vi "Class to Variant.vi"(8 "error in (no error)":errorcluster, 10 "Data in":variant, 11 "Run VI Node in":refnum<class "Run VI Node.lvclass">) -> (0 "error out":errorcluster, 1 "Serialized Object Name":string, 2 "Data":variant, 3 "Run VI Node out":refnum<class "Run VI Node.lvclass">)   [LabVIEW 2014, in "Run VI Node.lvclass"]
uses:
  Run VI Node.lvclass
  Shared/Controls/Run VI - STYP.ctl
  Run VI Node.lvclass/Run VI Node.ctl
  Classes/Build Job/Build Job.lvclass
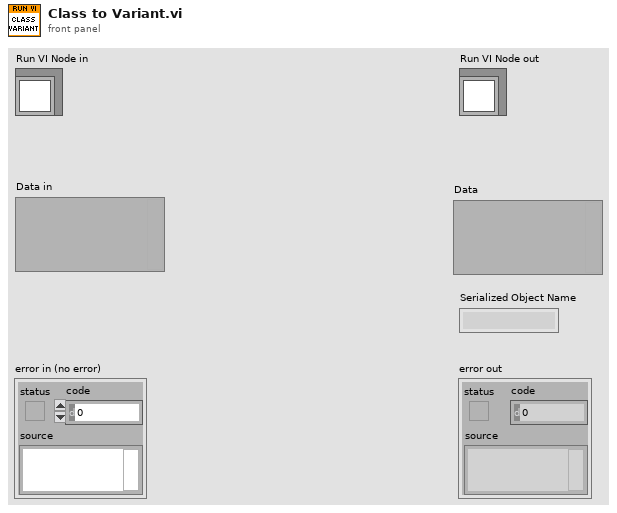
[diagram p1: front panel]
types:
  T1 = typedef "Run VI - STYP.ctl" = cluster{"Executor_Number":string, "VI_Path":string, "Wait_Until_Done":bool}
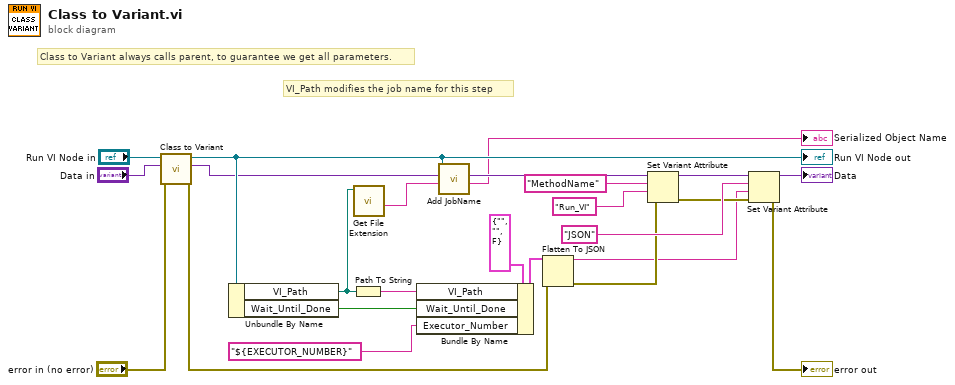
[diagram p0: block diagram]
diagram:
  # "VI_Path modifies the job name for this step"
  # "Class to Variant always calls parent, to guarantee we get all parameters."
  n1 = call-parent "Class to Variant.vi"("error in (no error)"="error in (no error)", "Data in"="Data in", "Build Job in"="Run VI Node in") -> ("error out"=w8:errorcluster, "Data Out"=w5:variant, "Build Job out"=w6:refnum<class "Run VI Node.lvclass">)  [unwired: 5 in, 1 out]
  "Run VI Node out" <- w6
  n2 = Unbundle By Name(w6) -> ("VI_Path"=w3:path, "Wait_Until_Done"=w18:bool)
  n3 = Path To String(path=w3) -> (string=w17:string)
  n4 = call <vilib>:"Get File Extension.vi"("file"=w3) -> ("filename without extension"=w2:string)  [unwired: 7 in, 3 out]
  n5 = Bundle By Name(cluster=T1 {"Executor_Number"="", "VI_Path"="", "Wait_Until_Done"=FALSE} ("Run VI"), "VI_Path"=w17, "Wait_Until_Done"=w18, "Executor_Number"="${EXECUTOR_NUMBER}") -> (w21:T1)
  n6 = call "Add JobName.vi"("Job Target"=w2, "Data in"=w5, "Build Job in"=w6) -> ("Job Name"=→"Serialized Object Name":string, "Data Out"=w4:variant)  [unwired: 7 in]
  n7 = Flatten To JSON(anything=w21, error in (no error)=w8) -> (JSON string=w9:string, 11:w11:errorcluster)  [unwired: 1 in]
  n8 = Set Variant Attribute(Variant=w4, name="MethodName", value="Run_VI", error in=w11) -> (Variant out=w13:variant, error out=w10:errorcluster)  [unwired: 1 out]
  n9 = Set Variant Attribute(Variant=w13, name="JSON" ("Name"), value=w9, error in=w10) -> (Variant out=→"Data":variant, error out=→"error out":errorcluster)  [unwired: 1 out]
